vi "Add Route.vi"(8 "error in (no error)":errorcluster, 9 "Navbar Page? (F)":bool, 10 "Endpoint":string, 11 "Path":string) -> (0 "error out":errorcluster)   [LabVIEW 2021, in "HttpServer.lvlib"]
uses:
  HttpServer.lvlib
  TypeDefs/Action.ctl
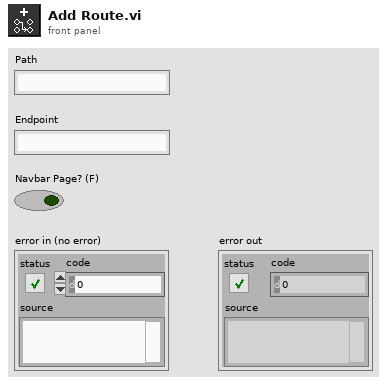
[diagram p1: front panel]
types:
  T1 = typedef "HttpServer.lvlib/Action.ctl" = enum8{"noop", "add", "get", "set", "remove"}
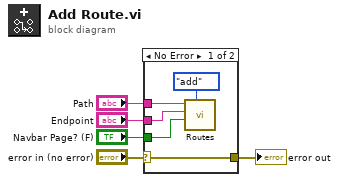
[diagram p0: block diagram]
diagram:
  n1 = case shown="No Error" "error in (no error)" {
    selector: "error in (no error)" -> [w7 w11]
    tunnel: "Path" -> [w9 _]
    tunnel: "Endpoint" -> [w8 _]
    tunnel: [w7 w11] -> w3
    tunnel: "Navbar Page? (F)" -> [w6 _]
    frame No Error {
      n2 = call "Routes.vi"("Action"=Action."add", "Navbar Page? (F)"=w6, "Endpoint in"=w8, "Path"=w9) -> ()  [unwired: 4 in, 4 out]
    }
    frame Error {
    }
  }
  "error out" <- w3
